vi "merge_Retentive Timer On.vi"   [LabVIEW 2017, in "NI_FunctionBlockMergeVIs.lvlib"]
doc: "A timer that counts up to <B>preset time (ms)</B> while <B>enable</B> is TRUE. When enable is FALSE, this function block retains the <B>accumulated time (ms)</B> value. When <B>accumulated time (ms)</B> reaches <B>preset time (ms)</B>, <B>done</B> returns TRUE until reset, but <B>accumulated time (ms)</B> continues to increment while <B>enable</B> is TRUE until reset."
uses:
  <vilib>/functionblocks/NI_FunctionBlockMergeVIs.lvlib
  <vilib>/functionblocks/FB Core/FB Core.xnode
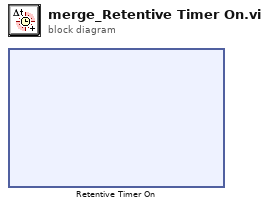
[diagram p0: block diagram]
diagram:
  n1 = xnode "Retentive Timer On"() -> ()  [unwired: 4 in, 3 out]
